vi "BETA - 0.1 - Motor Go To - David G.vi"(0 "Encoder Value":dbl=18000.0 format="%#_13g", 1 "Go To":dbl=18000.0 format="%#_13g", 3 "Speed":dbl=1.0 min=-1.0 max=1.0 format="%#_13g", 4 "Default Neutral Speed":dbl=1.0 min=-1.0 max=1.0 format="%#_13g", 5 "Button":bool=TRUE, 9 "Margin (Nullable)":dbl=18000.0 format="%#_13g") -> (8 "Output Neutral Speed":dbl=18000.0 format="%#_13g")   [LabVIEW 2018]
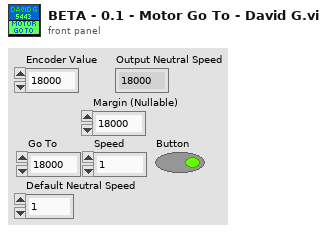
[diagram p1: front panel]
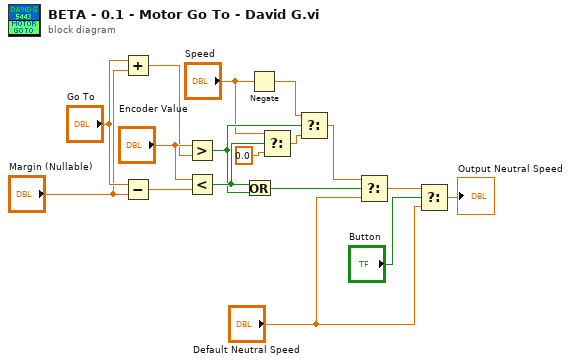
[diagram p0: block diagram]
diagram:
  n1 = Add(x="Go To", y="Margin (Nullable)") -> (x+y=w3:dbl)
  n2 = Subtract(x="Go To", y="Margin (Nullable)") -> (x-y=w4:dbl)
  n3 = Greater?(x="Encoder Value", y=w3) -> (0:w12:bool)
  n4 = Less?(x="Encoder Value", y=w4) -> (x < y?=w16:bool)
  n5 = Or(x=w16, y=w12) -> (x .or. y?=w11:bool)
  n6 = Negate(x="Speed") -> (-x=w8:dbl)
  n7 = Select(t="Speed", s=w16, f=0.0) -> (s? t:f=w14:dbl)
  n8 = Select(t=w8, s=w12, f=w14) -> (s? t:f=w13:dbl)
  n9 = Select(t=w13, s=w11, f="Default Neutral Speed") -> (s? t:f=w17:dbl)
  n10 = Select(t=w17, s="Button", f="Default Neutral Speed") -> (s? t:f=→"Output Neutral Speed":dbl)
